vi "MeasureFastBreakN.vi"(0 ".NET Refnum in":refnum<k24>, 1 ".NET Refnum":refnum<k24>, 2 "Junction Name":string, 5 "MaxVoltage":dbl, 7 "appended path":path, 12 "new file path (Not A Path if cancelled)":path, 13 "UiDefinition":T1, 14 "Function":string) -> (15 "error out":errorcluster)   [LabVIEW 2020]
uses:
  C:/Users/User/Desktop/Automation/CurrentVersion/LabviewDXFViewer/bin/Release/LabviewDXFViewer.exe
  LabviewDXFViewer/bin/Release/LabviewDXFViewer.exe
  UIReferences.ctl
  <vilib>/Utility/file.llb/Write Delimited Spreadsheet (DBL).vi
  <vilib>/Utility/file.llb/Write Delimited Spreadsheet (string).vi
panel:
  in  "CurrentPositionIndex":i32
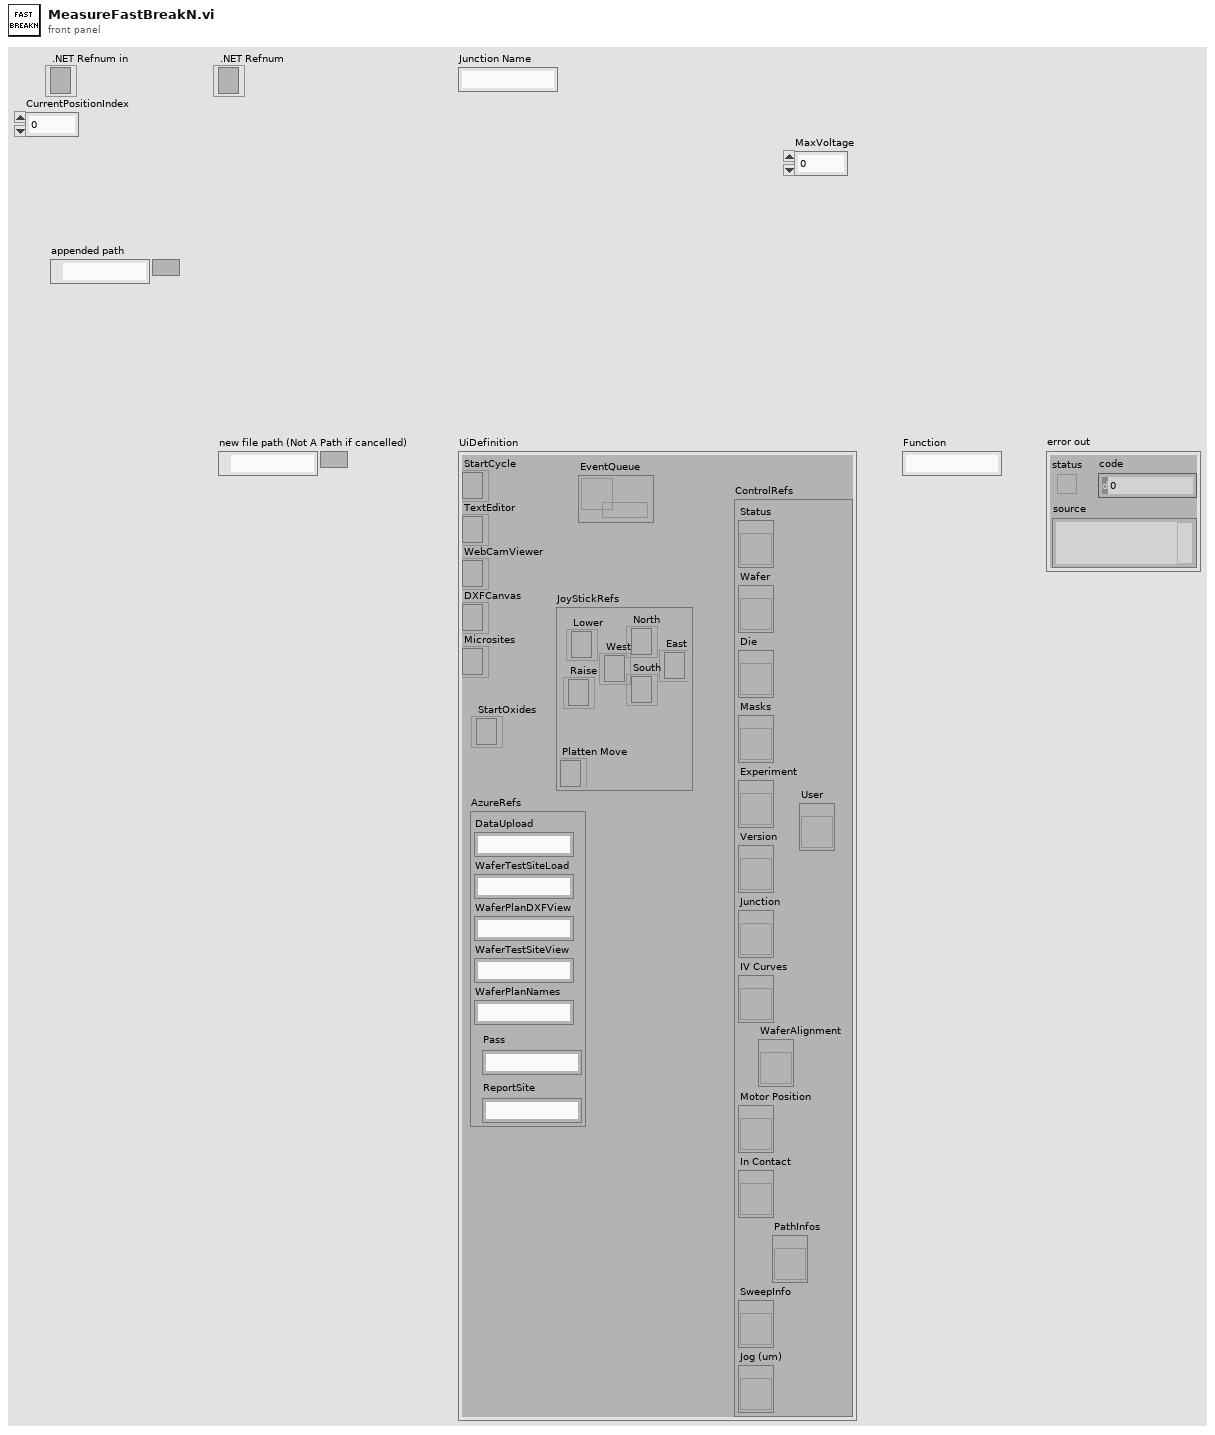
[diagram p1: front panel]
types:
  T1 = typedef "UIReferences.ctl" = cluster{"StartCycle":refnum<k24>, "TextEditor":refnum<k24>, "WebCamViewer":refnum<k24>, "DXFCanvas":refnum<k24>, "Microsites":refnum<k24>, "JoyStickRefs":cluster{"North":refnum<k24>, "Lower":refnum<k24>, "Raise":refnum<k24>, "Platten Move":refnum<k24>, "West":refnum<k24>, "East":refnum<k24>, "South":refnum<k24>}, "AzureRefs":cluster{"DataUpload":string, "WaferTestSiteLoad":string, "WaferPlanDXFView":string, "WaferTestSiteView":string, "WaferPlanNames":string, "Pass":string, "ReportSite":string}, "ControlRefs":cluster{"Status":refnum<vi>, "Wafer":refnum<vi>, "Die":refnum<vi>, "Masks":refnum<vi>, "Experiment":refnum<vi>, "Version":refnum<vi>, "Junction":refnum<vi>, "IV Curves":refnum<vi>, "Motor Position":refnum<vi>, "In Contact":refnum<vi>, "SweepInfo":refnum<vi>, "Jog (um)":refnum<vi>, "PathInfos":refnum<vi>, "User":refnum<vi>, "WaferAlignment":refnum<vi>}, "EventQueue":refnum<queue>, "StartOxides":refnum<k24>}
  T2 = cluster{"Current Range":dbl, "Source Measure Unit Channel (0: Channel A)":i32, "Waveform":waveform(dbl), "VISA resource name":refnum<visa-resource-name>, "CodeText":string}
  T3 = typedef "CapacitanceInfos.ctl" = cluster{"Conductance":dbl, "CapacitanceIV":dbl, "Intercept":dbl, "CapacitanceSW":dbl, "Sum":dbl, "CapacitanceInfos":T4[], "CapacitancePhase":dbl, "dC/dV":dbl, "Function":string, "OtherInfo":dbl[][]}
  T4 = typedef "CapacitanceRecord.ctl" = cluster{"Freq":dbl, "Vpp":dbl, "PhaseS":dbl, "Irms":dbl, "PhaseC":dbl, "Theta":dbl, "VDrive":dbl, "Capacitance":dbl, "Other":dbl}
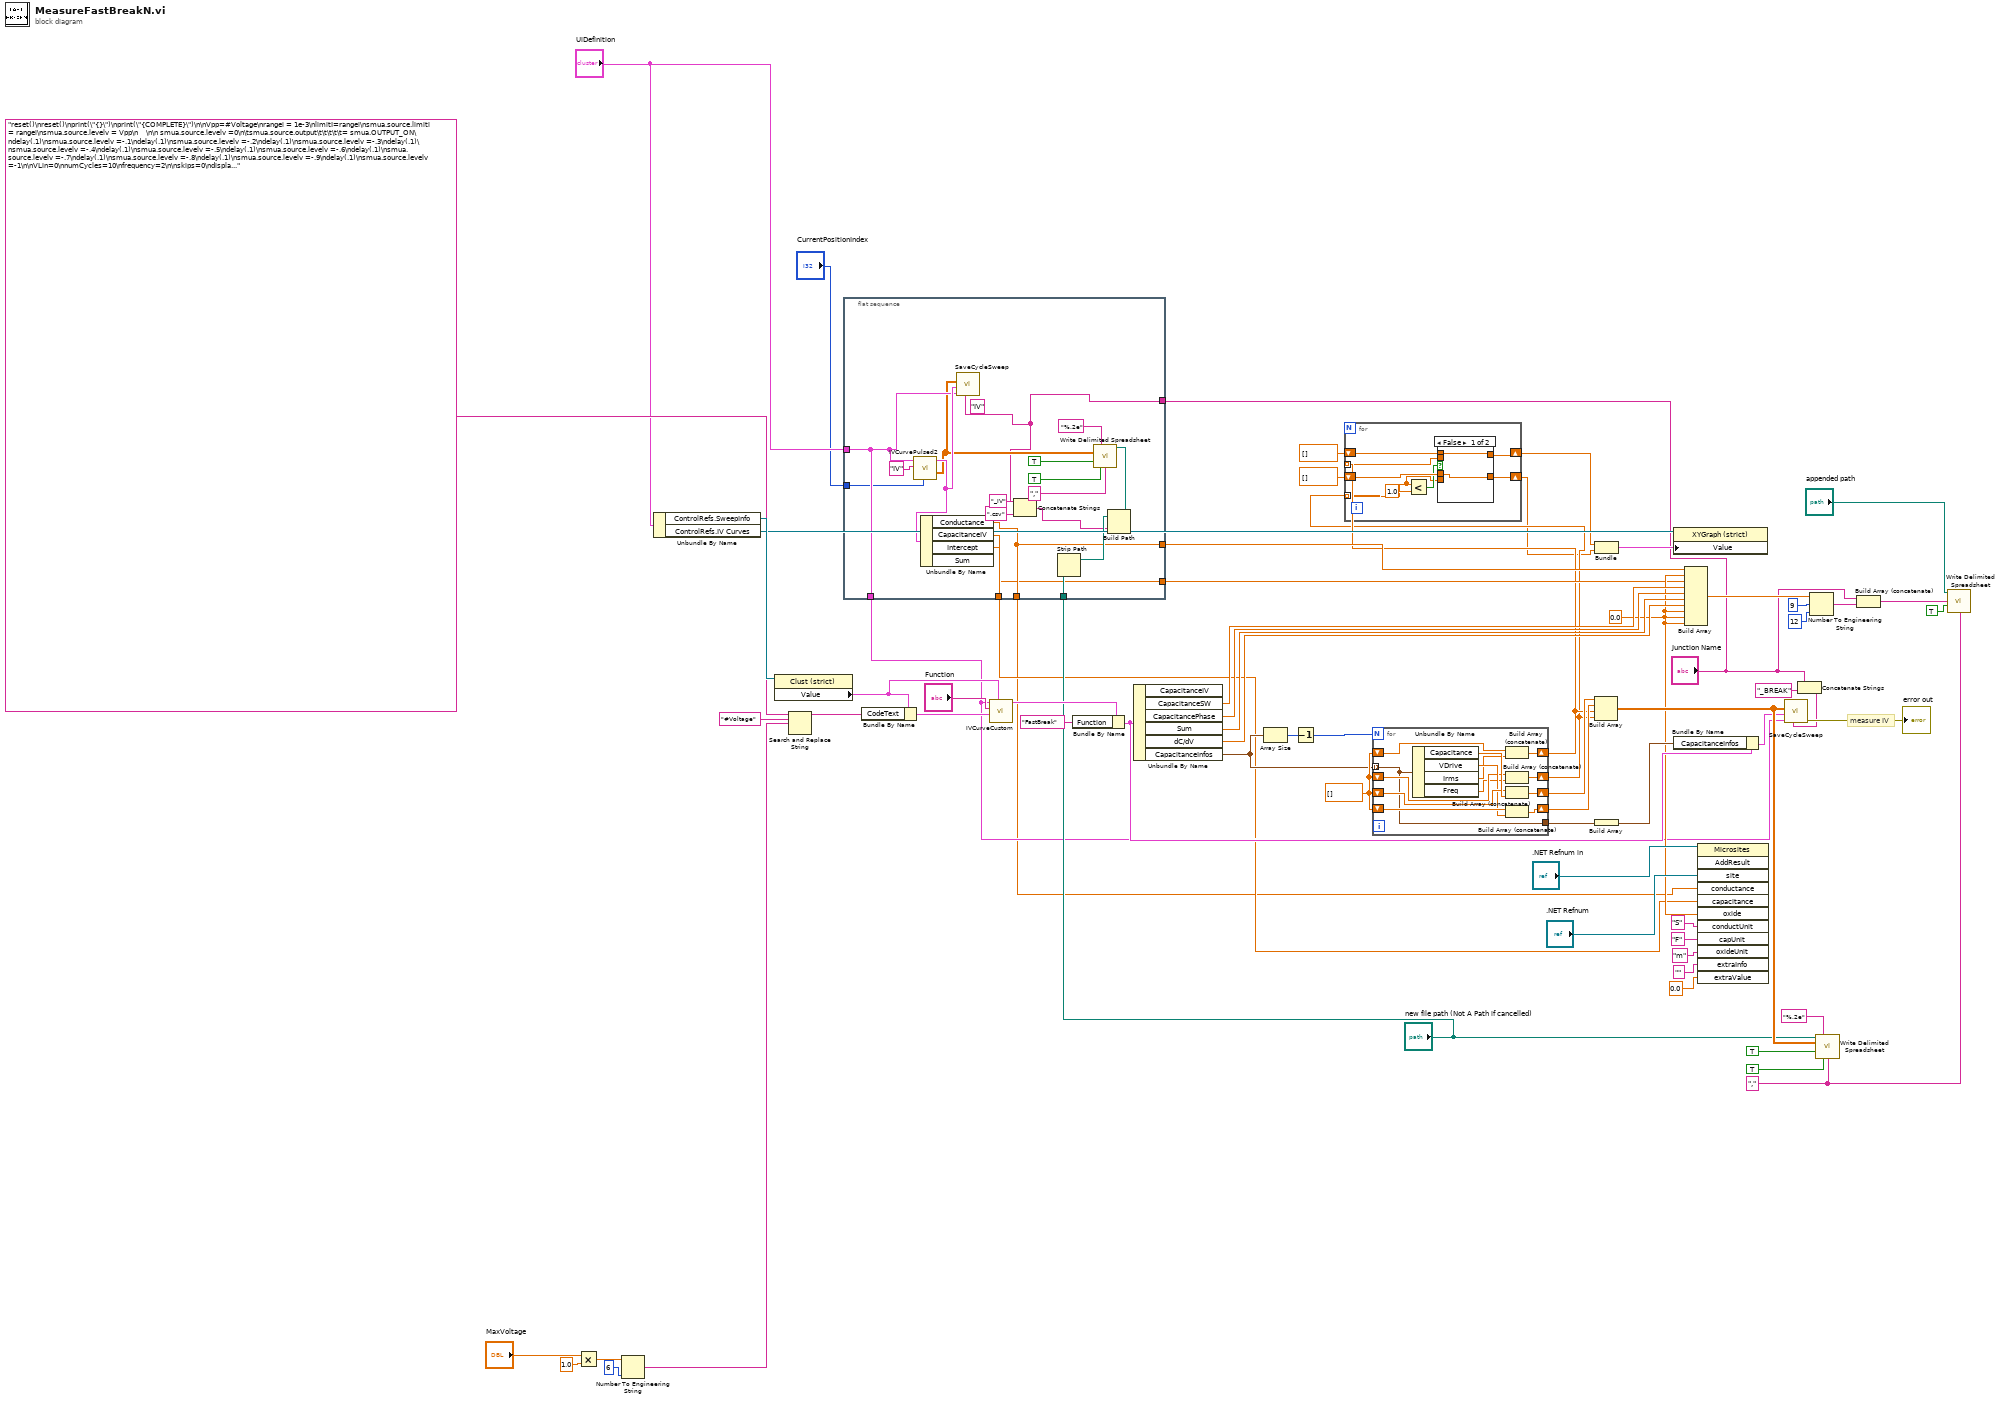
[diagram p0: block diagram]
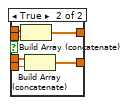
[diagram p2: hidden frame]
diagram:
  w41 = dbl[] []
  w21 = 0.0 ("element")
  w48 = "," ("delimiter (\\t)")
  # "measure IV"
  n1 = Multiply(x="MaxVoltage", y=1.0) -> (x*y=w28:dbl)
  n2 = Number To Engineering String(2:i16 6 ("precision (6)"), 4:w28) -> (0:w26:string)  [unwired: 2 in]
  n3 = Unbundle By Name("UiDefinition") -> ("ControlRefs.SweepInfo"=w46:refnum<vi>, "ControlRefs.IV Curves"=w42:refnum<vi>)
  n4 = property class="Clust (strict)"(reference=w46) -> ("Value"=w29:T2)  [unwired: 1 in, 2 out]
  n5 = Search and Replace String(input string="reset()\nreset()\nprint(\"{}\")\nprint(\"{COMPLETE}\")\n\nVpp=#Voltage\nrangei = 1e-3\nlimitI=rangei\nsmua.source.limiti = rangei\nsmua.source.levelv = Vpp\n    \n\n smua.source.levelv =0\n\tsmua.source.output\t\t\t\t\t= smua.OUTPUT_ON\ndelay(.1)\nsmua.source.levelv =-.1\ndelay(.1)\nsmua.source.levelv =-.2\ndelay(.1)\nsmua.source.levelv =-.3\ndelay(.1)\nsmua.source.levelv =-.4\ndelay(.1)\nsmua.source.levelv =-.5\ndelay(.1)\nsmua.source.levelv =-.6\ndelay(.1)\nsmua.source.levelv =-.7\ndelay(.1)\nsmua.source.levelv =-.8\ndelay(.1)\nsmua.source.levelv =-.9\ndelay(.1)\nsmua.source.levelv =-1\n\nVLin=0\nnumCycles=10\nfrequency=2\n\nskips=0\ndisplay=1\n\n\n\tlocal COMPLETE = \"{COMPLETE}\"\n\t-- Generate the source values\n\n\tlocal sourceValues\t\t= {} \n\tlocal pointsPerCycle\t= 60 / frequency\n\tlocal pointsPer60 = 1\n\tlocal numDataPoints\t\t= pointsPerCycle * numCycles\n\n\n\tp=(Vpp+1)/numDataPoints\n    for i = 1, numDataPoints do\n        sourceValues[i] =(i-1)*p-1\n      \n    end\n\n\t-- Configure the SMU ranges\n\tsmua.reset()\n\tsmua.source.settling\t\t= smua.SETTLE_FAST_POLARITY\n\tsmua.source.autorangev\t\t= smua.AUTORANGE_OFF\n\tsmua.source.autorangei\t\t= smua.AUTORANGE_OFF\nsmua.source.rangev\t\t\t= 10\n smua.source.limitv\t\t= 10\n\tsmua.source.delay\t\t\t= 0\n\tsmua.source.limiti\t\t\t=1e-3\n\n\tsmua.measure.autorangev\t\t= smua.AUTORANGE_OFF\n\tsmua.measure.autorangei\t\t= smua.AUTORANGE_OFF\n\tsmua.measure.autozero\t\t= smua.AUTOZERO_OFF\n\tsmua.measure.delay\t\t\t= 0\n\tsmua.measure.delayfactor    = 1\n\tsmua.measure.analogfilter   = 0\n\n\t-- Voltage will be measured on the same range as the source range\n\tsmua.measure.rangei\t\t\t=limitI\n\tsmua.measure.nplc\t\t\t=1\n\n\t-- Prepare the Reading Buffers\n\tsmua.nvbuffer1.clear()\n\tsmua.nvbuffer1.collecttimestamps\t= 1\n\tsmua.nvbuffer2.clear()\n\tsmua.nvbuffer2.collecttimestamps\t= 1\n\n\t-- Configure the trigger model\n\t--============================\n\t\n\t-- Timer 1 controls the time between source points\n\ttrigger.timer[1].delay = (1 / 60)\n\ttrigger.timer[1].passthrough = true\n\ttrigger.timer[1].stimulus = smua.trigger.ARMED_EVENT_ID\n\ttrigger.timer[1].count = numDataPoints - 1\n\n\t-- Configure the SMU trigger model\n\tsmua.trigger.source.listv(sourceValues)\n\tsmua.trigger.source.limiti\t\t= limitI\n\tsmua.trigger.measure.action\t\t= smua.ENABLE\n\tsmua.trigger.measure.iv(smua.nvbuffer1, smua.nvbuffer2)\n\tsmua.trigger.endpulse.action\t= smua.SOURCE_HOLD\n\tsmua.trigger.endsweep.action\t= smua.SOURCE_IDLE\n\tsmua.trigger.count\t\t\t\t= numDataPoints\n\tsmua.trigger.arm.stimulus\t\t= 0\n\tsmua.trigger.source.stimulus\t= trigger.timer[1].EVENT_ID\n\tsmua.trigger.measure.stimulus\t= 0\n\tsmua.trigger.endpulse.stimulus\t= 0\n\tsmua.trigger.source.action\t\t= smua.ENABLE\n\t-- Ready to begin the test\n\n\tsmua.source.output\t\t\t\t\t= smua.OUTPUT_ON\n\t-- Start the trigger model execution\n\tsmua.trigger.initiate()\n\t-- Wait until the sweep has completed\n\twaitcomplete()\n\tsmua.source.output\t\t\t\t\t= smua.OUTPUT_OFF\n\n\t-- Print the data back to the Console in tabular format\n\nfor x=1, smua.nvbuffer2.n,pointsPer60 do\n     if (smua.nvbuffer2[x]>.008) then\n         print(smua.nvbuffer1[x], 1, 1.0/60,smua.nvbuffer1.timestamps[x] ,0 , 0, sourceValues[x],smua.nvbuffer2[x],0)\n     end\n\tend\n\nprint(\"{COMPLETE}\")\n\nsmua.source.output = smua.OUTPUT_OFF" ("CodeText"), search string="#Voltage", replace string=w26) -> (result string=w33:string)  [unwired: 5 in, 3 out]
  n6 = flat-sequence {
    tunnel: "new file path (Not A Path if cancelled)" -> [w82]
    tunnel: "UiDefinition" -> [w75]
    tunnel: [w75] -> w15
    tunnel: [w79] -> w14
    tunnel: [w78] -> w13
    tunnel: [w78] -> w12
    tunnel: [w77] -> w11
    tunnel: "Junction Name" -> [w70]
    tunnel: "CurrentPositionIndex" -> [w69]
    frame #0 {
      (unwired) "IV" ("string")
      n7 = call "IVCurvePulsed2.vi"("CurrentPositionIndex"=w69, "Program"="IV", "UiDefinition"=w75) -> ("appended array"=w74:dbl[][], "InfoCluster"=w76:T3)  [unwired: 7 in]
      n8 = Unbundle By Name(w76) -> ("Conductance"=w78:dbl, "CapacitanceIV"=w79:dbl, "Intercept"=w77:dbl)  [unwired: 1 out]
      n9 = call "SaveCycleSweep.vi"("JunctionName"=w70, "UiDefinition 2"=w75, "InfoCluster"=w76, "appended array"=w74) -> ()  [unwired: 7 in, 1 out]
      n10 = Concatenate Strings(w70, "_IV" ("string"), ".csv" ("string")) -> (w72:string)
      n11 = Strip Path(path=w82) -> (stripped path=w80:path)  [unwired: 1 out]
      n12 = Build Path(base path=w80, name or relative path=w72) -> (appended path=w81:path)
      n13 = call-poly <vilib>:"Write Delimited Spreadsheet.vi"("file path (dialog if empty)"=w81, "format (%.3f)"="%.2e", "2D data"=w74, "append to file? (new file:F)"=TRUE, "transpose? (no:F)"=TRUE, "delimiter (\\t)"="," ("delimiter (\\t)")) -> ()  [unwired: 8 in, 2 out]
    }
  }
  n14 = Bundle By Name(cluster=w29, "CodeText"=w33) -> (w32:T2)
  n15 = call "IVCurveCustom.vi"("OriginalSweepInfo"=w29, "SweepInfo"=w32, "Program"="Function", "UiDefinition"=w15) -> ("InfoCluster"=w30:T3)  [unwired: 6 in, 1 out]
  n16 = Bundle By Name(cluster=w30, "Function"="FastBreak") -> (w45:T3)
  n17 = Unbundle By Name(w45) -> ("CapacitanceSW"=w61:dbl, "CapacitancePhase"=w62:dbl, "Sum"=w59:dbl, "dC/dV"=w60:dbl, "CapacitanceInfos"=w20:T4[])  [unwired: 1 out]
  n18 = Array Size(array=w20) -> (size(s)=w19:i32)
  n19 = Decrement(x=w19) -> (x-1=w18:i32)
  n20 = for {
    N: w18 -> [_]
    tunnel: w20 -> [w88] mode=indexing
    shift-right: [w100] -> w38
    shift-left: w41 -> [w98]
    shift-right: [w97] -> w40
    shift-left: w41 -> [w96]
    shift-right: [w93] -> w9
    shift-left: w41 -> [w94]
    shift-right: [w91] -> w8
    shift-left: w41 -> [w92]
    tunnel: [w88] -> w23
    n21 = Unbundle By Name(w88) -> ("Capacitance"=w99:dbl, "VDrive"=w95:dbl, "Irms"=w90:dbl, "Freq"=w89:dbl)
    n22 = Build Array (concatenate)(w94, w90) -> (w93:dbl[])
    n23 = Build Array (concatenate)(w92, w89) -> (w91:dbl[])
    n24 = Build Array (concatenate)(w98, w99) -> (w100:dbl[])
    n25 = Build Array (concatenate)(w96, w95) -> (w97:dbl[])
  }
  n26 = for {
    tunnel: w9 -> [w101] mode=indexing
    tunnel: w8 -> [w102] mode=indexing
    shift-right: [w108] -> w4
    shift-left: dbl[] [] -> [w106]
    shift-right: [w107] -> w5
    shift-left: dbl[] [] -> [w105]
    n27 = Less?(x=w102, y=1.0) -> (x < y?=w103:bool)
    n28 = case shown="False" w103 {
      tunnel: [w109 w116] -> w108
      tunnel: [w110 w115] -> w107
      tunnel: w106 -> [w109 w114]
      tunnel: w105 -> [w110 w113]
      tunnel: w102 -> [_ w112]
      tunnel: w101 -> [_ w111]
      frame False {
      }
      frame True {
        n29 = Build Array (concatenate)(w113, w111) -> (w115:dbl[])
        n30 = Build Array (concatenate)(w114, w112) -> (w116:dbl[])
      }
    }
  }
  n31 = Build Array(w38, w40, w9, w8) -> (w39:dbl[][])
  n32 = Bundle(w5, w4) -> (w37:cluster{dbl[], dbl[]})  [unwired: 1 in]
  n33 = Build Array(w23) -> (w22:T4[])
  n34 = property class="XYGraph (strict)"(reference=w42, "Value"=w37) -> ()  [unwired: 1 in, 2 out]
  n35 = Bundle By Name(cluster=w45, "CapacitanceInfos"=w22) -> (w24:T3)
  n36 = Build Array(w12, w21, w11, w61, w62, w59, w60, w21, w21, w21) -> (w58:dbl[])
  n37 = invoke class="Microsites" method="AddResult"(reference=".NET Refnum in", "site"=".NET Refnum", "conductance"=w13, "capacitance"=w14, "oxide"=w21, "conductUnit"="S", "capUnit"="F", "oxideUnit"="m" ("interceptUnit"), "extraInfo"="", "extraValue"=0.0) -> ()  [unwired: 2 in, 12 out]
  n38 = Concatenate Strings("Junction Name", "_BREAK" ("string")) -> (w3:string)
  n39 = call "SaveCycleSweep.vi"("JunctionName"=w3, "UiDefinition 2"=w15, "InfoCluster"=w24, "appended array"=w39) -> ("error out"=→"error out":errorcluster)  [unwired: 7 in]
  n40 = Number To Engineering String(2:i16 12 ("precision (6)"), 3:i16 9 ("width (-)"), 4:w58) -> (0:w51:string[])  [unwired: 1 in]
  n41 = call-poly <vilib>:"Write Delimited Spreadsheet.vi"("file path (dialog if empty)"="new file path (Not A Path if cancelled)", "format (%.3f)"="%.2e", "2D data"=w39, "append to file? (new file:F)"=TRUE, "transpose? (no:F)"=TRUE, "delimiter (\\t)"=w48) -> ()  [unwired: 8 in, 2 out]
  n42 = Build Array (concatenate)("Junction Name", w51) -> (w53:string[])
  n43 = call-poly <vilib>:"Write Delimited Spreadsheet.vi"("file path (dialog if empty)"="appended path", "1D data"=w53, "append to file? (new file:F)"=TRUE, "delimiter (\\t)"=w48) -> ()  [unwired: 10 in, 2 out]
